vi "Execute action2.vi"(8 "error in (no error)":errorcluster, 10 "Action":string, 11 "Class path":path) -> (0 "error out":errorcluster)   [LabVIEW 2021]
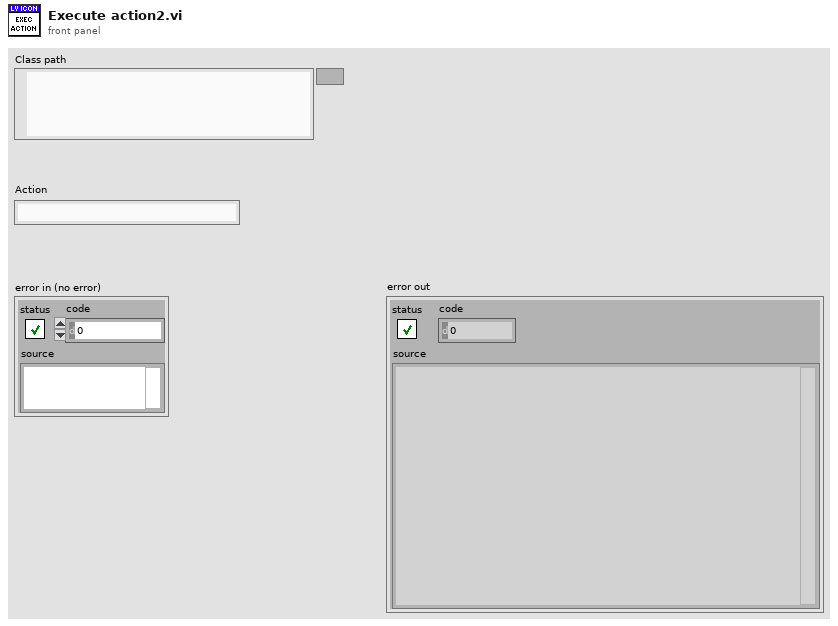
[diagram p1: front panel]
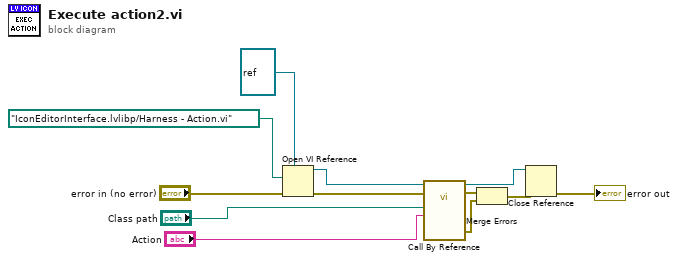
[diagram p0: block diagram]
diagram:
  n1 = Open VI Reference(type specifier VI Refnum (for type only)=refnum<vi> refnum, vi path=path "IconEditorInterface.lvlibp/Harness - Action.vi", error in (no error)="error in (no error)") -> (vi reference=w10:refnum<vi>, error out=w11:errorcluster)  [unwired: 3 in]
  n2 = call-by-ref "?"(reference=w10, error in=w11, "Action"="Action", "Class"="Class path") -> (reference out=w5:refnum<vi>, error out=w3:errorcluster, 0:"error out"=w2:errorcluster)  [unwired: 9 in]
  n3 = Merge Errors(w3, w2) -> (w1:errorcluster)
  n4 = Close Reference(reference=w5, error in (no error)=w1) -> (error out=→"error out":errorcluster)
